vi "OnTempStabilized Ext VI.vi"(0 "Finished":bool, 1 "AVS Data":T1) -> ()   [LabVIEW 2019]
panel:
  # "Do not rename or delete\nthis control"
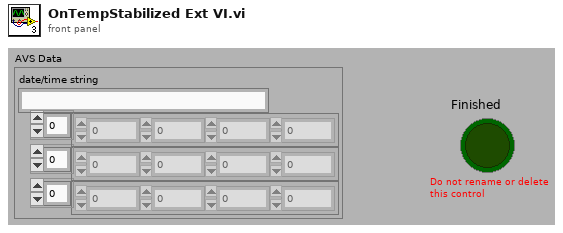
[diagram p1: front panel]
types:
  T1 = cluster{"date/time string":string, dbl[], dbl[], dbl[]}
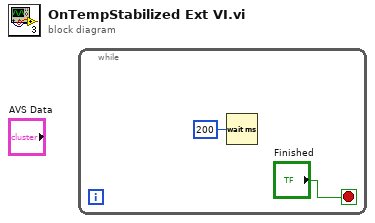
[diagram p0: block diagram]
diagram:
  n1 = while {
    stop <- "Finished" stop-if-true
    n2 = Wait (ms)(milliseconds to wait=u32 200) -> ()  [unwired: 1 out]
  }
